vi "4.0 EMGtoOMG LIVE troubleshooting.vi"() -> ()   [LabVIEW 2018]
uses:
  <vilib>/express/express analysis/Spectral/Block/exnSpectralBlock spectral measurements power poly.vi
  <vilib>/express/express analysis/Spectral/Block/exnSpectralBlock spectral measurements power DDT.vi
  <vilib>/express/express analysis/Spectral/XNode/ExpressSpectralMeasurementsBlockNode.xnode
panel:
  out "Output 22-43":string[](array[string])
  out "seq175-209":dbl[](array[numeric])
  out "seq140-174":dbl[](array[numeric])
  out "seq105-139":dbl[](array[numeric])
  in  "file path (use dialog) 2":path
  in  "Numeric 3":dbl=0.05 format="%#_13g"
  in  "Numeric 2":dbl=0.05 format="%#_13g"
  in  "Numeric":dbl=0.05 format="%#_13g"
  in  "rate":dbl=5000.0
  in  "sample size":i32=5000
  out "RMS 3":dbl
  out "RMS 2":dbl
  out "RMS":dbl
  out "return value":string
  out "Output 00-21":string[](array[string])
  out "c":i32[](array[numeric])
  out "state":dbl[](array[numeric])
  out "charSearch":dbl[](array[numeric])
  out "seq70-104":dbl[](array[numeric])
  out "seq35-69":dbl[](array[numeric])
  out "setID":dbl[](array[numeric])
  out "seq00-34":dbl[](array[numeric])
  in  "stop":bool
  in  "module path":path
  # "1-1-3     3 (x8) \"G\"     1-2-1     3 (x4) \"o\"     2     1-1-2     3 (x2) \"b\"     1-2-1     3 (x1) \"l\"     1-2-2     3 (x5) \"u\"     1-1-2     3 (x5) \"e\"     2     1-3-1     3 (x4) \"!\"     1-1-1     2     3 (x2)     2     1"
  # "1-1-1 -> Edit text\n\n1-1-2 -> Set 1 ' abcdeABCDE'\n\n1-1-3 -> Set 2 ' fghijkFGHIJK' \n\n1-2-1 -> Set 3 ' lmnopLMNOP' \n\n1-2-2 -> Set 4 ' qrstuQRSTU'\n\n1-2-3 -> Set 5 ' vwxyzVWXYZ' \n\n1-3-1 -> Set 6 ' .,?!>\\'\\\"@#&_-+=' \n\n1-3-2 -> Set 7 ' ()[]<>/\\|%^*~'\n\n1-3-3 -> Set 8 ' 0123456789'"
  # "To the right of the three signals is a \"state\" indicator. \n\nState 1 - \"Unknown\" \n-Program is  waiting for a 1 to start building setID.\n-While in State 1, 2s and 3s don't do anything. \n- Enter a 1 to change to State 2 and begin recording a setID.\n\nState 2 - \"Find\"\n-Program stores next two inputs into setID.\n-The ID can be seen in the setID indicator. The first the numbers is the ID of the set, the 4th number is the associated number of the set (1-8)\n-An ID of 1-1-1 is invalid, and this will change the state back to state 1. \n-All other sets are valid and change state to State 3\n\nState 3 - \"Nav\"\n-Program cycles through and selects a chosen character in a set\n-Repeating 3s will cycle forward through a set, currently selected character is in {}\n-2 will enter the selected character and stay in the current set, and reset the cycle\n-1 will enter the selected character and acts as the first digit in a new setID, and changes to State 2\n\nUse the following sequence as practice:\n2332-121-3-113-3333-122-33333333333-3333-1\n\n2332 does nothing\n121 chooses Set 3\n3 cycles through Set 3\n113 selects character and chooses Set 2\n3333 cycles through Set 2\n122 selects character and chooses Set 4\n33333333333 (eleven 3s) cycles completely through Set 4\n3333 cycles through set 4\n1 selects character"
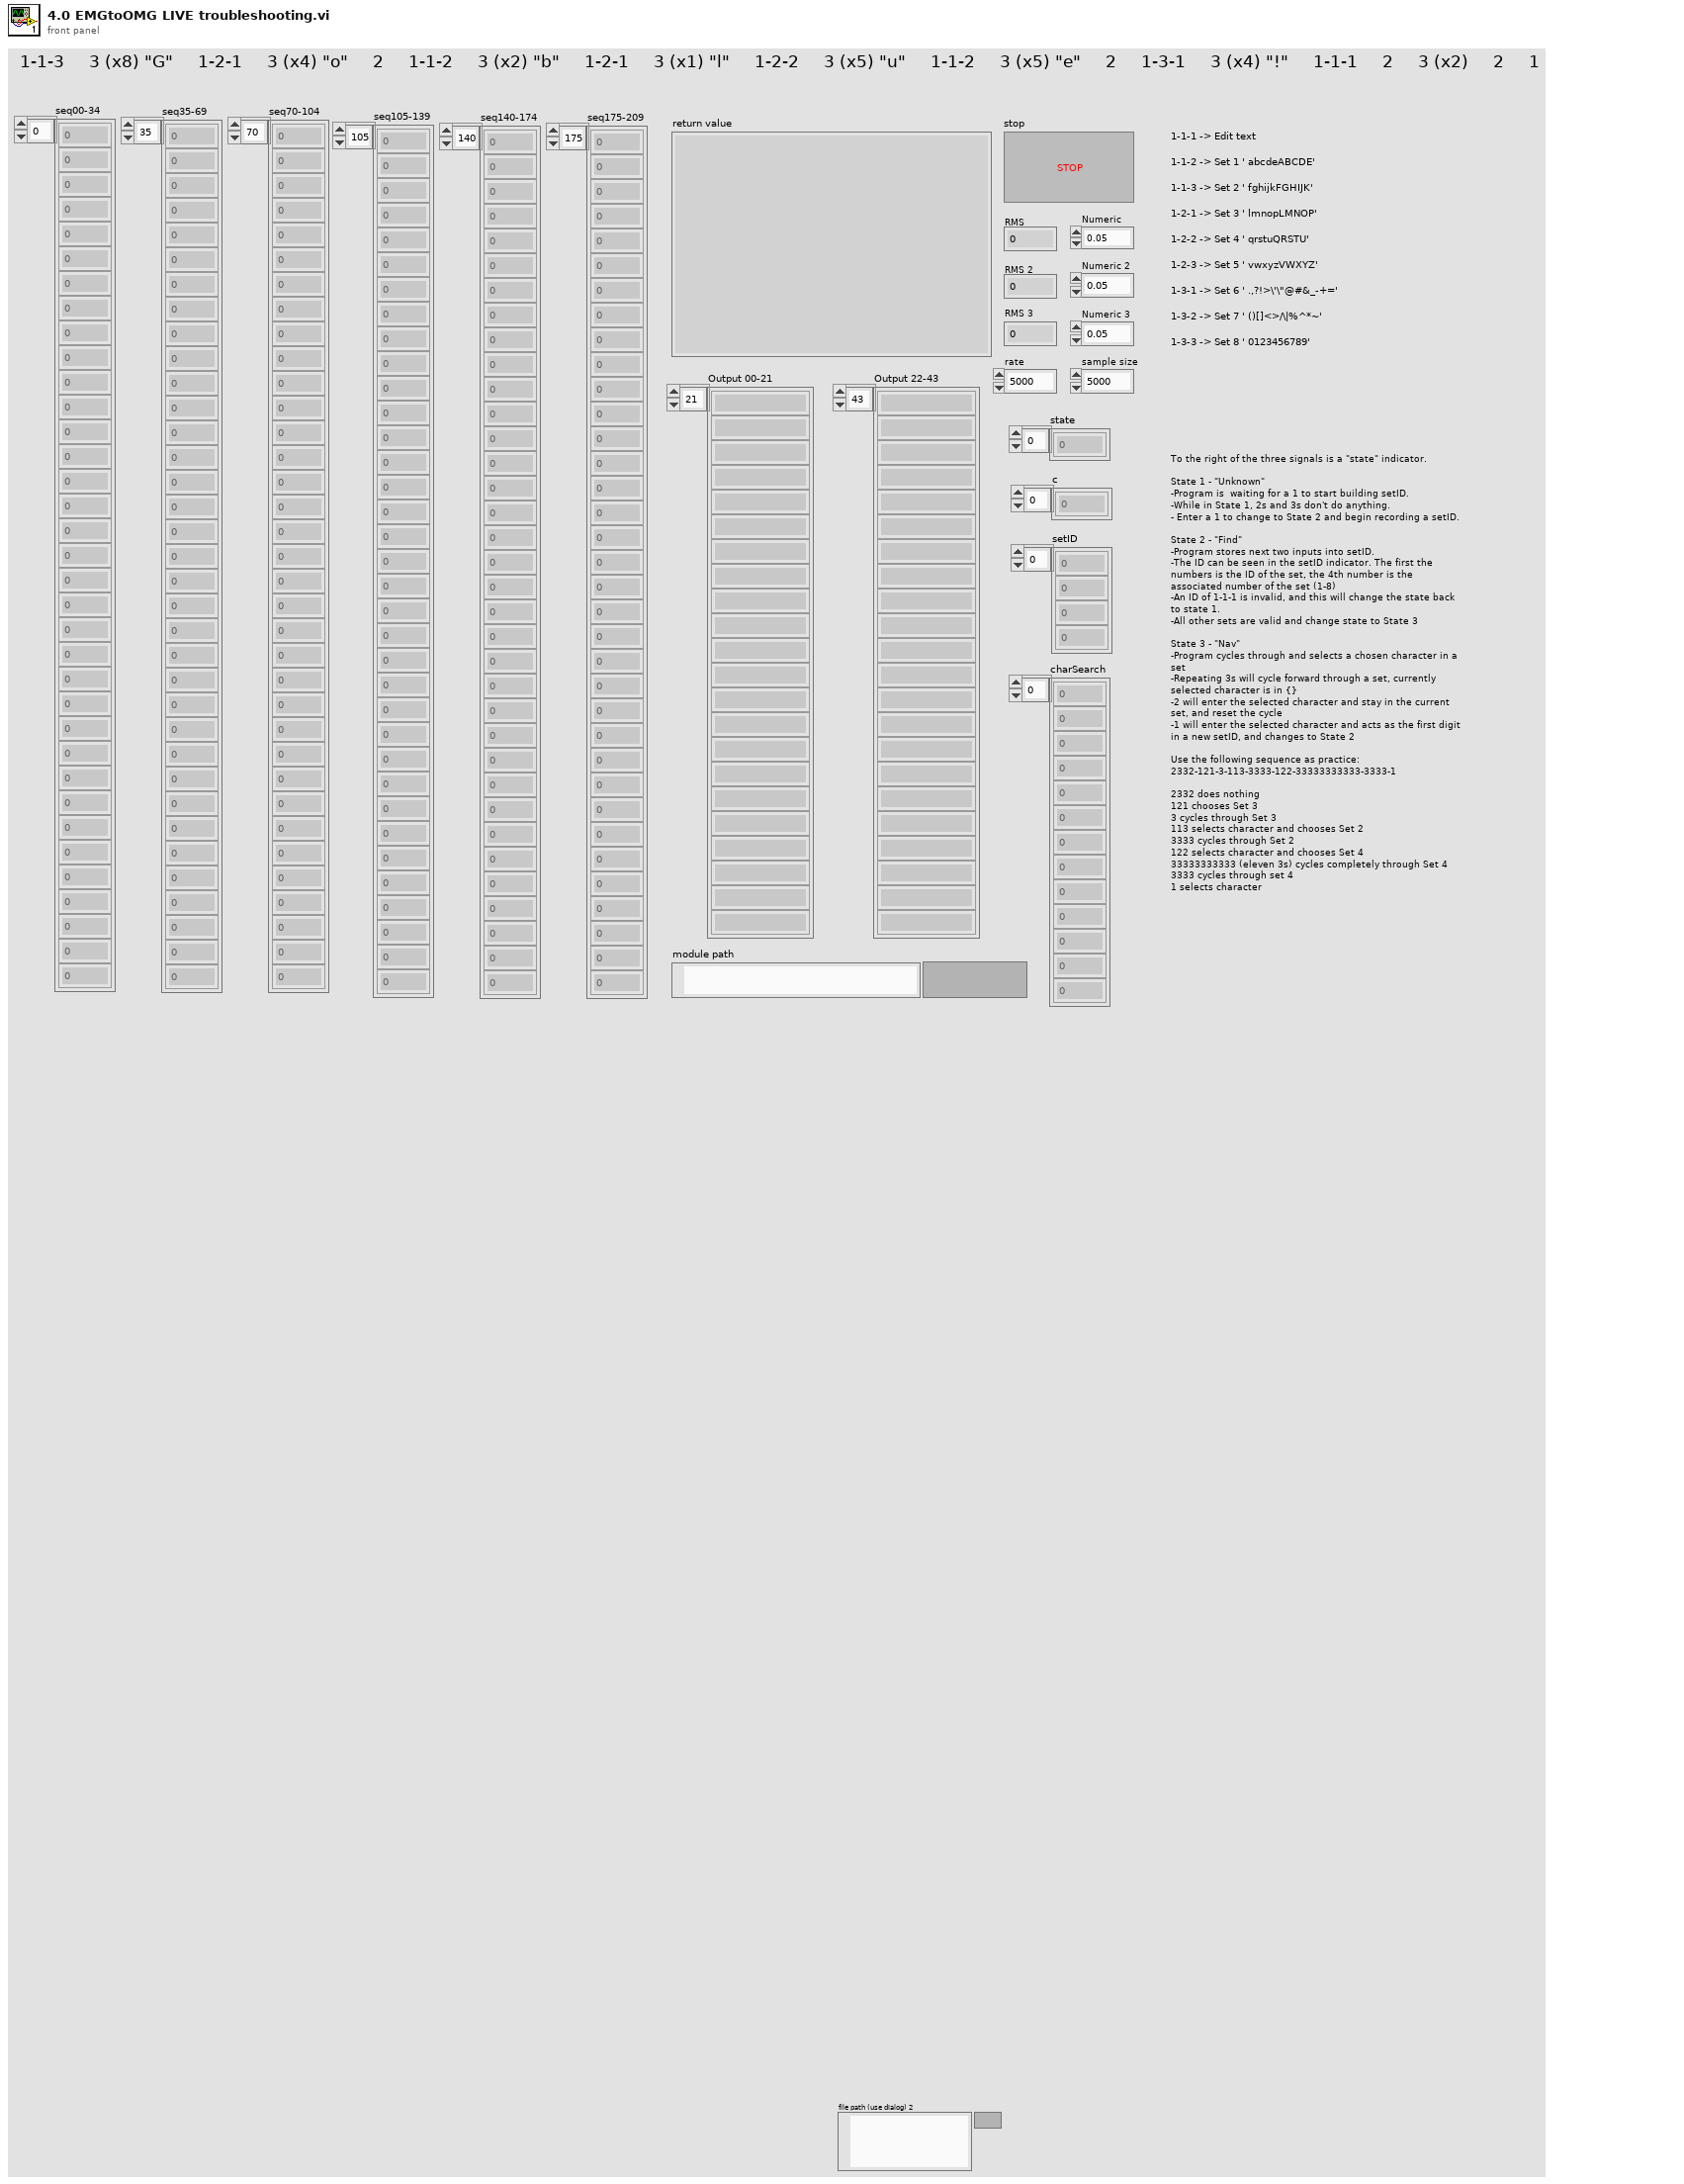
[diagram p1: front panel]
types:
  T1 = enum16{"open", "replace", "create", "open or create", "replace or create", "replace or create with confirmation"}
  T2 = cluster{"averaging mode":u16, "weighting mode":u16, "number of averages":u32}
  T3 = cluster{"dB On (F)":bool, "unwrap phase (F)":bool, "convert to degree (F)":bool}
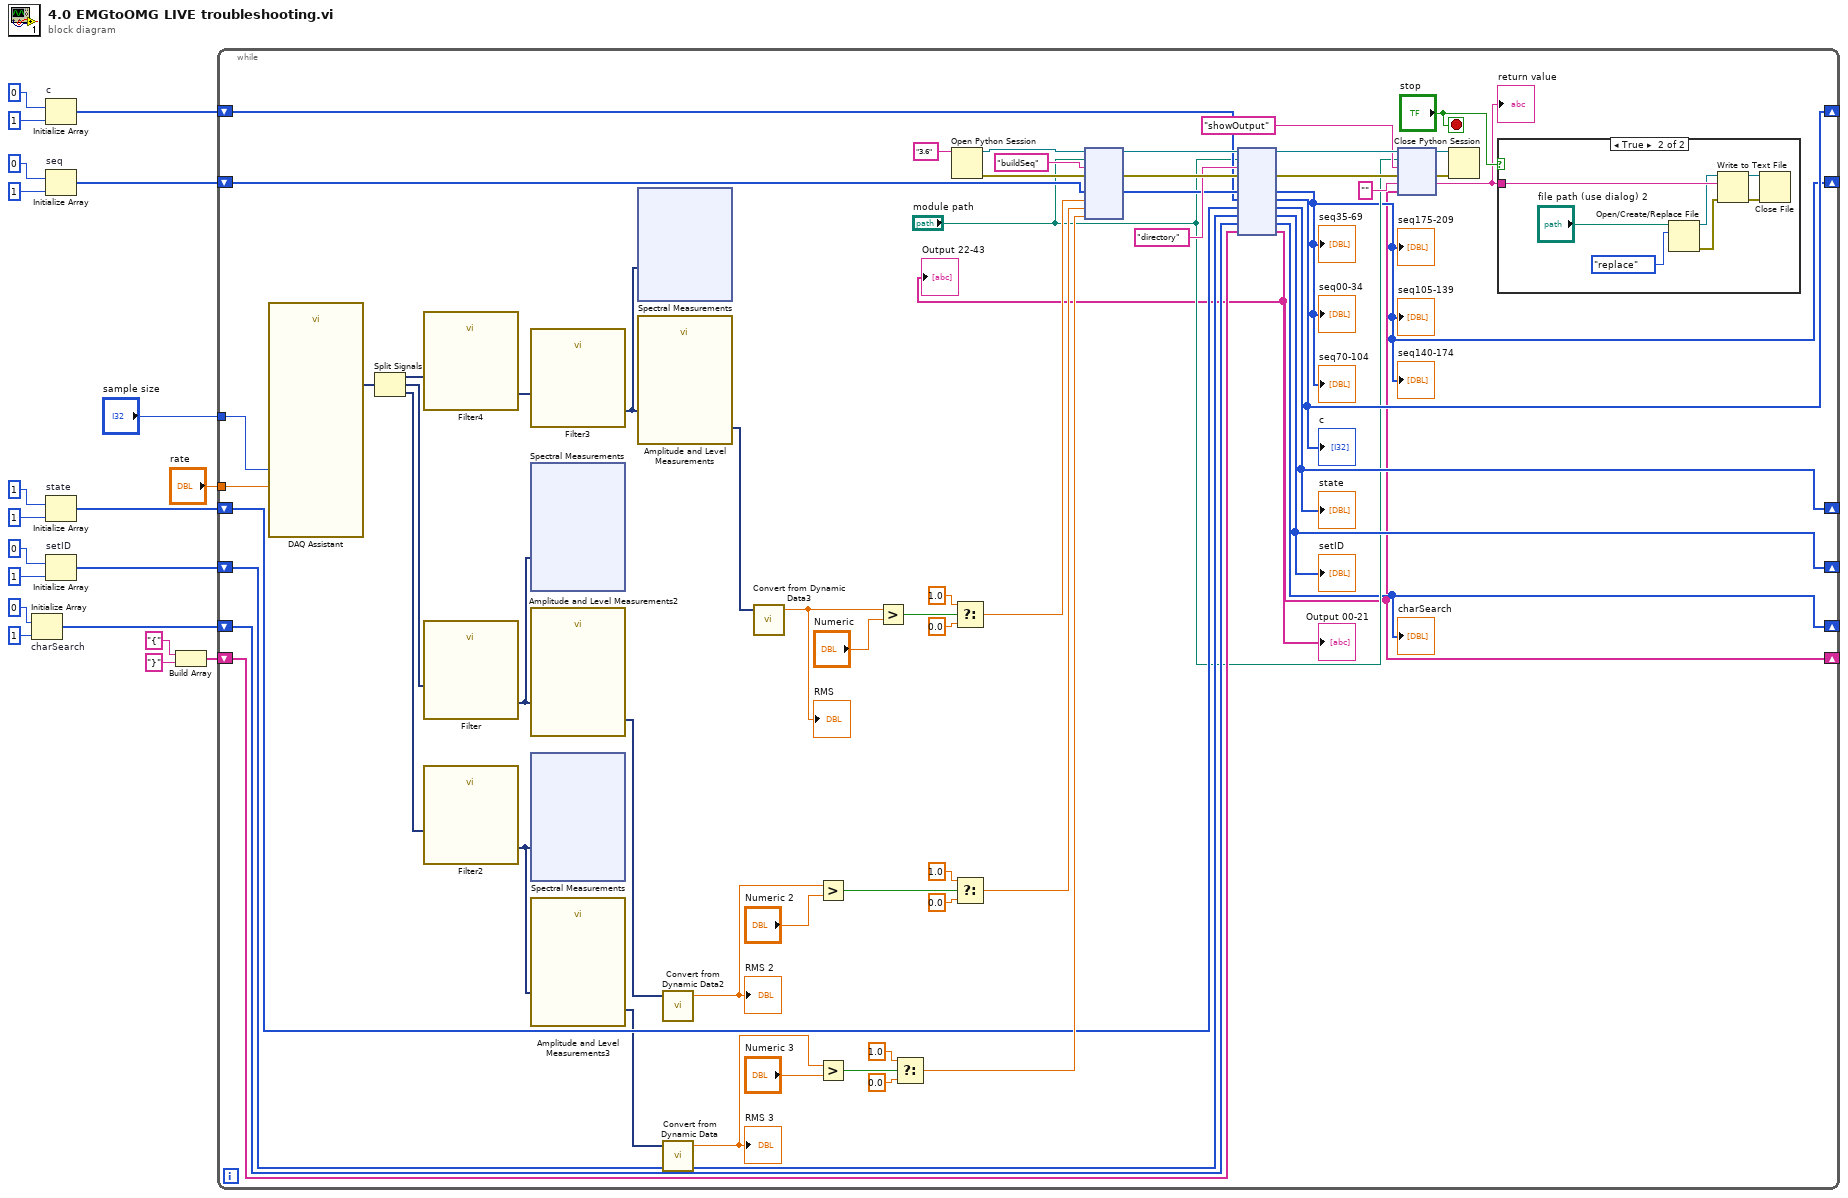
[diagram p0: block diagram]
diagram:
  n1 = Initialize Array "charSearch"(0, 1 ("dimension size")) -> (w15:i32[])
  n2 = Initialize Array "c"(0, 1 ("dimension size")) -> (w13:i32[])
  n3 = Initialize Array "seq"(0, 1 ("dimension size")) -> (w20:i32[])
  n4 = Initialize Array "state"(1, 1 ("dimension size")) -> (w10:i32[])
  n5 = Initialize Array "setID"(0, 1 ("dimension size")) -> (w16:i32[])
  n6 = Build Array("{", "}") -> (w7:string[])
  n7 = while {
    shift-right: [w22] -> _
    shift-left: w20 -> [w73]
    shift-right: [w59] -> _
    shift-left: w16 -> [w62]
    shift-right: [w47] -> _
    shift-left: w15 -> [w61]
    shift-right: [w21] -> _
    shift-left: w7 -> [w60]
    shift-right: [w57] -> _
    shift-left: w10 -> [w58]
    shift-right: [w55] -> _
    shift-left: w13 -> [w56]
    tunnel: "sample size" -> [w26]
    tunnel: "rate" -> [w25]
    stop <- "stop" stop-if-true
    n8 = call "DAQ Assistant"("rate"=w25, "number of samples"=w26) -> ("data"=w44:dynamicdata)  [unwired: 15 in, 2 out]
    n9 = Split Signals(w44) -> (w40:dynamicdata, w43:dynamicdata, w42:dynamicdata)  [unwired: 3 in]
    n10 = call "Filter4"("Signal"=w40) -> ("Filtered Signal"=w39:dynamicdata)  [unwired: 9 in, 1 out]
    n11 = call "Filter"("Signal"=w43) -> ("Filtered Signal"=w46:dynamicdata)  [unwired: 9 in, 1 out]
    n12 = call "Filter2"("Signal"=w42) -> ("Filtered Signal"=w45:dynamicdata)  [unwired: 9 in, 1 out]
    n13 = call "Filter3"("Signal"=w39) -> ("Filtered Signal"=w41:dynamicdata)  [unwired: 9 in, 1 out]
    n14 = xnode "Spectral Measurements"("Signals"=w46) -> ()  [unwired: 1 in, 2 out]
    n15 = call "Amplitude and Level Measurements2"("Signals"=w46) -> ("RMS"=w36:dynamicdata)  [unwired: 13 in, 1 out]
    n16 = xnode "Spectral Measurements"("Signals"=w45) -> ()  [unwired: 1 in, 2 out]
    n17 = call "Amplitude and Level Measurements3"("Signals"=w45) -> ("RMS"=w38:dynamicdata)  [unwired: 13 in, 1 out]
    n18 = xnode "Spectral Measurements"("Signals"=w41) -> ()  [unwired: 1 in, 2 out]
    n19 = call "Amplitude and Level Measurements"("Signals"=w41) -> ("RMS"=w34:dynamicdata)  [unwired: 13 in, 1 out]
    n20 = call "Convert from Dynamic Data2"("Dynamic Data Type"=w36) -> ("Scalar"=w30:dbl)  [unwired: 3 in]
    "RMS 2" <- w30
    n21 = call "Convert from Dynamic Data"("Dynamic Data Type"=w38) -> ("Scalar"=w32:dbl)  [unwired: 3 in]
    "RMS 3" <- w32
    n22 = call "Convert from Dynamic Data3"("Dynamic Data Type"=w34) -> ("Scalar"=w29:dbl)  [unwired: 3 in]
    "RMS" <- w29
    n23 = Greater?(x=w30, y="Numeric 2") -> (0:w28:bool)
    n24 = Greater?(x=w32, y="Numeric 3") -> (0:w31:bool)
    n25 = Greater?(x=w29, y="Numeric") -> (0:w27:bool)
    n26 = Select(t=1.0, s=w31, f=0.0) -> (s? t:f=w67:dbl)
    n27 = Open Python Session(python version="3.6" ("Python version")) -> (session out=w79:refnum<k35>, error out=w78:errorcluster)  [unwired: 2 in]
    n28 = Select(t=1.0, s=w27, f=0.0) -> (s? t:f=w76:dbl)
    n29 = Select(t=1.0, s=w28, f=0.0) -> (s? t:f=w68:dbl)
    n30 = node(w79, "module path", "buildSeq" ("function name"), w78, w73, w76, w68, w67) -> (w66:refnum<k35>, w65:errorcluster, w63:i32[])  [unwired: 5 in, 2 out]
    n31 = node(w66, "module path", "directory" ("function name"), w65, w63, w56, w58, w62, w61, w60) -> (w53:refnum<k35>, w51:errorcluster, w22:i32[], w55:i32[], w57:i32[], w59:i32[], w47:i32[], w21:string[])  [unwired: 2 in, 2 out]
    "seq00-34" <- w22
    "setID" <- w59
    "seq35-69" <- w22
    "seq70-104" <- w22
    "charSearch" <- w47
    "state" <- w57
    "c" <- w55
    "Output 00-21" <- w21
    "seq105-139" <- w22
    "seq140-174" <- w22
    "seq175-209" <- w22
    "Output 22-43" <- w21
    n32 = node(w53, "module path", "showOutput" ("function name"), w51, "", w21) -> (w52:refnum<k35>, w50:errorcluster, w23:string)  [unwired: 1 in, 2 out]
    "return value" <- w23
    n33 = Close Python Session(session in=w52, error in=w50) -> ()  [unwired: 1 out]
    n34 = case shown="True" "stop" {
      tunnel: w23 -> [_ w87]
      frame False {
      }
      frame True {
        n35 = Open/Create/Replace File(file path (use dialog)="file path (use dialog) 2", operation (0:open)=T1."replace") -> (refnum out=w83:refnum<file>, error out=w84:errorcluster)  [unwired: 4 in, 1 out]
        n36 = Write to Text File(file (use dialog)=w83, text=w87, error in=w84) -> (refnum out=w85:refnum<file>, error out=w86:errorcluster)  [unwired: 1 in, 1 out]
        n37 = Close File(refnum=w85, error in=w86) -> ()  [unwired: 2 out]
      }
    }
  }
